vi "Chassis_Create.vi"(9 "vAngular":dbl, 10 "vY":dbl, 11 "vX":dbl) -> (3 "CHASSIS":T1)   [LabVIEW 2019, in "PathExecution_Library.lvlib"]
uses:
  PathExecution_Library.lvlib
  CHASSIS.ctl
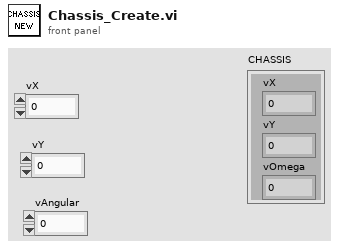
[diagram p1: front panel]
types:
  T1 = typedef "PathExecution_Library.lvlib/CHASSIS.ctl" = cluster{"vX":dbl, "vY":dbl, "vOmega":dbl}
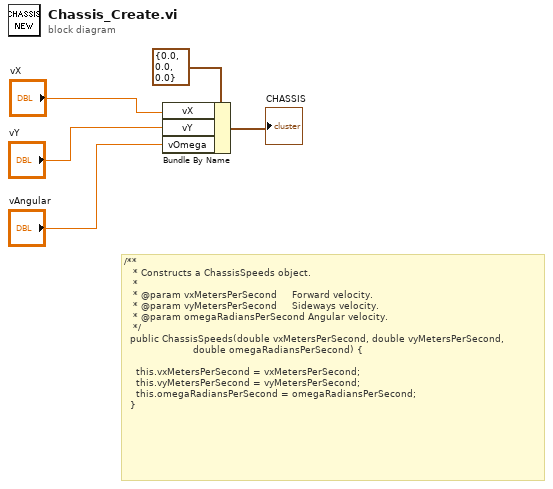
[diagram p0: block diagram]
diagram:
  # "/**\n   * Constructs a ChassisSpeeds object.\n   *\n   * @param vxMetersPerSecond     Forward velocity.\n   * @param vyMetersPerSecond     Sideways velocity.\n   * @param omegaRadiansPerSecond Angular velocity.\n   */\n  public ChassisSpeeds(double vxMetersPerSecond, double vyMetersPerSecond,\n                       double omegaRadiansPerSecond) {\n\n    this.vxMetersPerSecond = vxMetersPerSecond;\n    this.vyMetersPerSecond = vyMetersPerSecond;\n    this.omegaRadiansPerSecond = omegaRadiansPerSecond;\n  }"
  n1 = Bundle By Name(cluster=T1 {"vX"=0.0, "vY"=0.0, "vOmega"=0.0} ("CHASSIS"), "vX"="vX", "vY"="vY", "vOmega"="vAngular") -> (→"CHASSIS":T1)
